vi "Client Command.vi"(8 "error in (no error)":errorcluster, 9 "Context":variant, 10 "Message":string, 11 "Communications in":refnum<class "Communications.lvclass">) -> (0 "error out":errorcluster, 1 "Context out":variant, 3 "Communications out":refnum<class "Communications.lvclass">)   [LabVIEW 2019, in "Communications.lvclass"]
uses:
  Communications.lvclass
  C:/Program Files/National Instruments/LabVIEW 2019/vi.lib/ActorFramework/Actor/Actor.lvclass
  <vilib>/ActorFramework/Actor/Actor.lvclass/Actor.ctl
  Controllers/Application Controller Messages/Monitor Command Msg/Monitor Command Msg.lvclass/Monitor Command Msg.ctl
  <vilib>/ActorFramework/Message Enqueuer/Message Enqueuer.lvclass/Message Enqueuer.ctl
  <vilib>/ActorFramework/Message Enqueuer/Enqueue.vi
  Controllers/Application Controller Messages/Monitor Command Msg/Monitor Command Msg.lvclass
  C:/Program Files/National Instruments/LabVIEW 2019/vi.lib/ActorFramework/Message/Message.lvclass
  <vilib>/ActorFramework/Message Priority Queue/Priority Enqueue.vi
  <vilib>/ActorFramework/Actor/Actor.lvclass
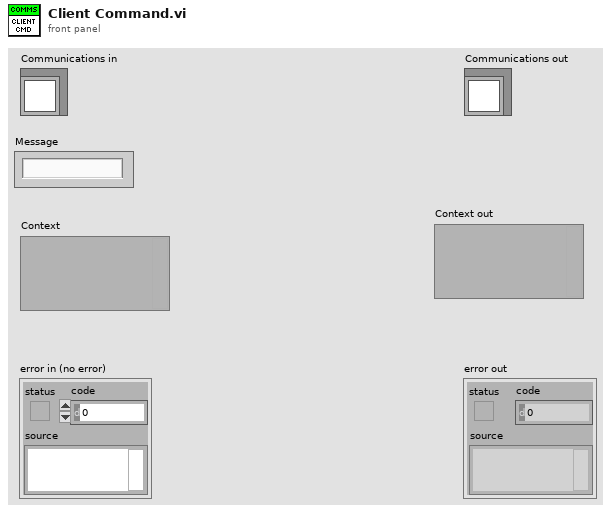
[diagram p1: front panel]
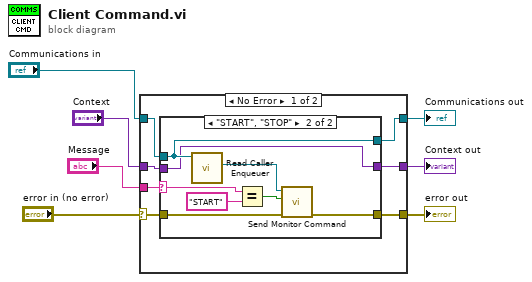
[diagram p0: block diagram]
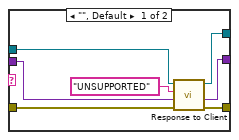
[diagram p2: hidden frame]
diagram:
  n1 = case shown="No Error" "error in (no error)" {
    selector: "error in (no error)" -> [w13 w32]
    tunnel: [w12 w32] -> w6
    tunnel: [w8 w31] -> w4
    tunnel: "Communications in" -> [w14 w31]
    tunnel: "Message" -> [w9 _]
    tunnel: "Context" -> [w11 w30]
    tunnel: [w10 w30] -> w1
    frame No Error {
      n2 = case shown="\"START\", \"STOP\"" w9 {
        selector: w9 -> [_ w24]
        tunnel: w14 -> [w19 w29]
        tunnel: w13 -> [w21 w27]
        tunnel: [w17 w25] -> w10
        tunnel: [w20 w26] -> w12
        tunnel: [w18 w29] -> w8
        tunnel: w11 -> [w15 w25]
        frame "", Default {
          n3 = call-dynamic "Response to Client.vi"("error in (no error)"=w21, "Context"=w15, "Message"="UNSUPPORTED", "Communications in"=w19) -> ("error out"=w20:errorcluster, "Context out"=w17:variant, "Communications out"=w18:refnum<class "Communications.lvclass">)  [unwired: 5 in]
        }
        frame "START", "STOP" {
          n4 = call <vilib>:"Read Caller Enqueuer.vi"("Actor"=w29) -> ("Caller Enqueuer"=w28:refnum<class "Message Enqueuer.lvclass">)  [unwired: 10 in]
          n5 = Equal?(x=w24, y="START") -> (x = y?=w22:bool)
          n6 = call "Send Monitor Command.vi"("error in (no error)"=w27, "StartStop"=w22, "Message Enqueuer"=w28) -> ("error out"=w26:errorcluster)  [unwired: 7 in, 1 out]
        }
      }
    }
    frame Error {
    }
  }
  "error out" <- w6
  "Communications out" <- w4
  "Context out" <- w1
